vi "Punto 1.vi"() -> ()   [LabVIEW 2020]
panel:
  in  "Operate fuction":bool
  out "C":dbl
  out "B":dbl
  out "A":dbl
  in  "Fuction:":string
  out "X value 1":dbl
  out "X value 2":dbl
  in  "Parar\naplicación":bool
  in  "Parar\naplicación":bool
  out "X value":dbl
  in  "Operate 4y^2-(2z/3)":bool
  in  "Operate 2y^3 + v(10z)":bool
  in  "Operate 44y - 21 z":bool
  in  "Operate 2y + 10z":bool
  in  "Z number":dbl
  in  "Y number":dbl
  # "This program was created by Juan Bermúdez from the Army Aviation School\nat the Aircraft Engineering of the assignature of Programation II"
  # "How to write the fuction?:\n1- First write all in lower case.\n2- Second, write every coefficient, even if this is 0 or 1.\n3- Third, write without spaces.\n4- Forth, write only the necesary things, coming up, some examples:\n\n- 1x^2+2x+3\n- 3x^2-0x+1\n- -4x^2+1x+0\n- -1x^2-10x-9\n The before examples are the correct way to write the fuction."
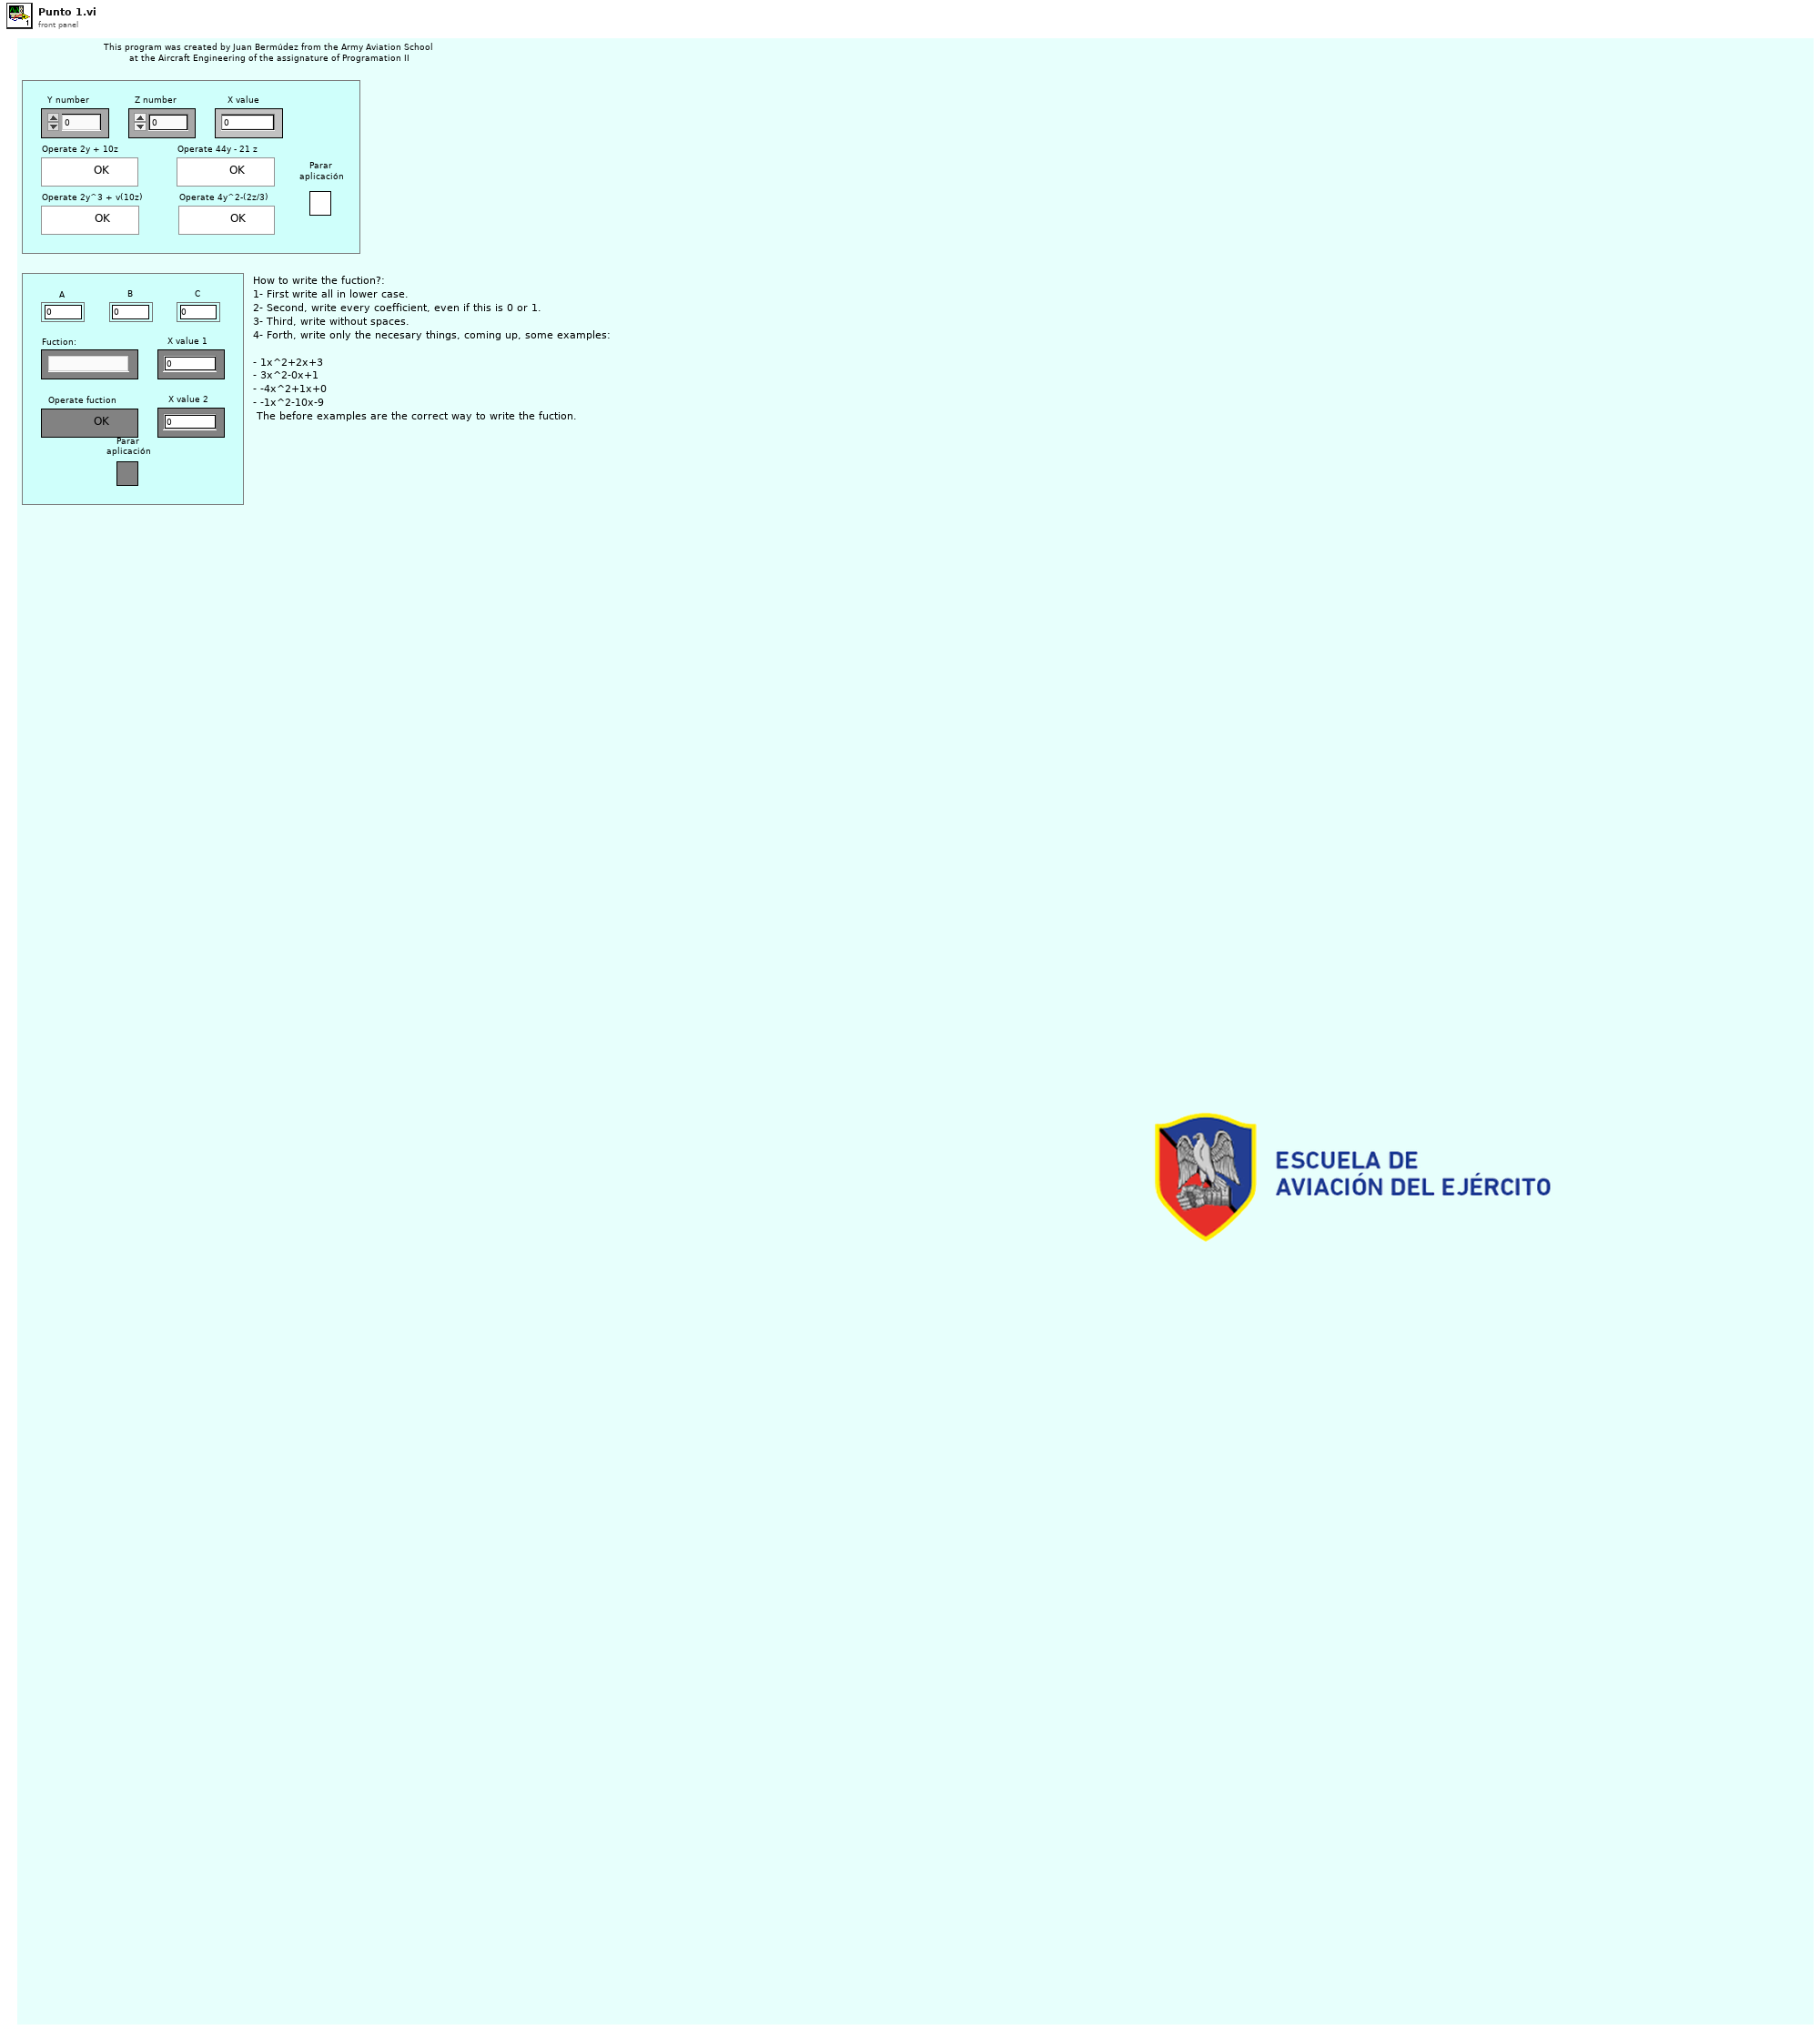
[diagram p1: front panel]
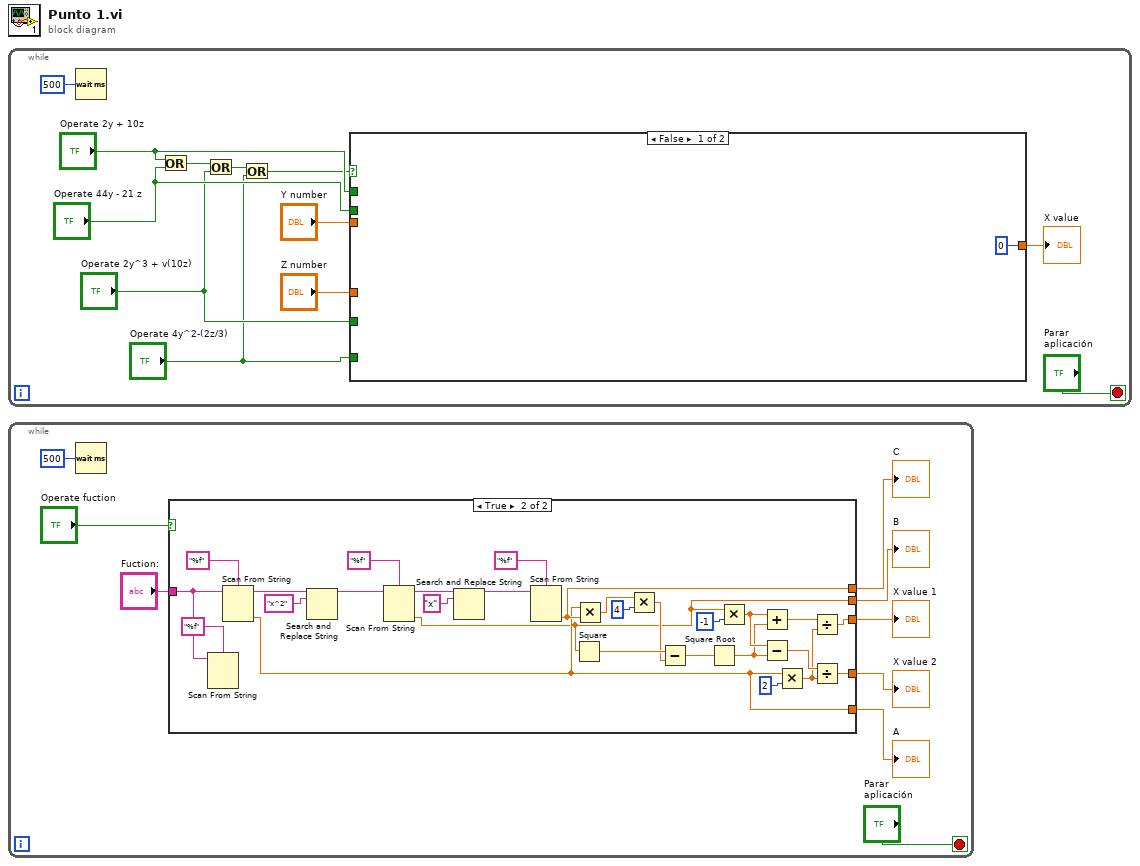
[diagram p0: block diagram]
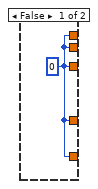
[diagram p2: hidden frame]
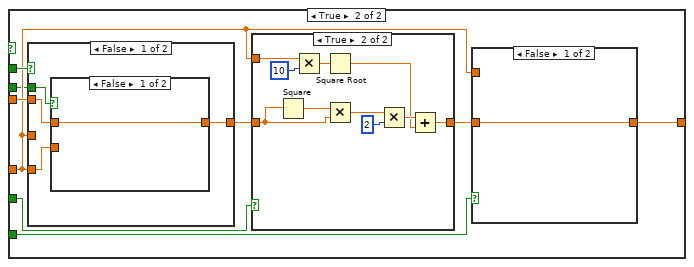
[diagram p3: hidden frame]
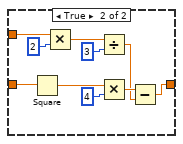
[diagram p4: hidden frame]
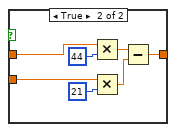
[diagram p6: hidden frame]
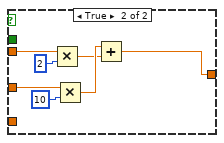
[diagram p7: hidden frame]
diagram:
  n1 = while {
    stop <- "Parar\naplicación" stop-if-true
    n2 = Wait (ms)(milliseconds to wait=500) -> ()  [unwired: 1 out]
    n3 = Or(x="Operate 2y + 10z", y="Operate 44y - 21 z") -> (x .or. y?=w5:bool)
    n4 = Or(x=w5, y="Operate 2y^3 + v(10z)") -> (x .or. y?=w3:bool)
    n5 = Or(x=w3, y="Operate 4y^2-(2z/3)") -> (x .or. y?=w1:bool)
    n6 = case shown="False" w1 {
      tunnel: "Operate 2y + 10z" -> [_ w22]
      tunnel: "Y number" -> [_ w21]
      tunnel: "Operate 2y^3 + v(10z)" -> [_ w20]
      tunnel: "Operate 4y^2-(2z/3)" -> [_ w19]
      tunnel: [0 w17] -> w11
      tunnel: "Z number" -> [_ w16]
      tunnel: "Operate 44y - 21 z" -> [_ w14]
      frame False {
      }
      frame True {
        n7 = case shown="False" w22 {
          tunnel: w16 -> [_ w61]
          tunnel: w21 -> [w46 w63]
          tunnel: w16 -> [w48 _]
          tunnel: [w47 w57] -> w15
          tunnel: w14 -> [w45 _]
          frame False {
            n8 = case shown="False" w45 {
              tunnel: w46 -> [w49 w56]
              tunnel: w48 -> [_ w54]
              tunnel: [w49 w50] -> w47
              frame False {
              }
              frame True {
                n9 = Multiply(x=w56, y=44) -> (x*y=w52:dbl)
                n10 = Multiply(x=w54, y=21) -> (x*y=w51:dbl)
                n11 = Subtract(x=w52, y=w51) -> (x-y=w50:dbl)
              }
            }
          }
          frame True {
            n12 = Multiply(x=w63, y=2) -> (x*y=w58:dbl)
            n13 = Multiply(x=w61, y=10) -> (x*y=w59:dbl)
            n14 = Add(x=w59, y=w58) -> (x+y=w57:dbl)
          }
        }
        n15 = case shown="True" w20 {
          tunnel: w15 -> [w34 w43]
          tunnel: w16 -> [_ w40]
          tunnel: [w34 w35] -> w18
          frame False {
          }
          frame True {
            n16 = Square(x=w43) -> (x^2=w44:dbl)
            n17 = Multiply(x=w40, y=10) -> (x*y=w38:dbl)
            n18 = Square Root(x=w38) -> (sqrt(x)=w36:dbl)
            n19 = Multiply(x=w44, y=w43) -> (x*y=w42:dbl)
            n20 = Multiply(x=w42, y=2) -> (x*y=w37:dbl)
            n21 = Add(x=w37, y=w36) -> (x+y=w35:dbl)
          }
        }
        n22 = case shown="False" w19 {
          tunnel: w18 -> [w23 w33]
          tunnel: w16 -> [_ w30]
          tunnel: [w23 w24] -> w17
          frame False {
          }
          frame True {
            n23 = Square(x=w33) -> (x^2=w32:dbl)
            n24 = Multiply(x=w30, y=2) -> (x*y=w28:dbl)
            n25 = Divide(x=w28, y=3) -> (x/y=w25:dbl)
            n26 = Multiply(x=w32, y=4) -> (x*y=w26:dbl)
            n27 = Subtract(x=w26, y=w25) -> (x-y=w24:dbl)
          }
        }
      }
    }
    "X value" <- w11
  }
  n28 = while {
    stop <- "Parar\naplicación" stop-if-true
    n29 = Wait (ms)(milliseconds to wait=500) -> ()  [unwired: 1 out]
    n30 = case shown="True" "Operate fuction" {
      tunnel: [w73 w89] -> w70
      tunnel: [w73 w88] -> w69
      tunnel: "Fuction:" -> [_ w75]
      tunnel: [w73 w78] -> w67
      tunnel: [w73 w77] -> w66
      tunnel: [w73 w76] -> w65
      frame False {
        w73 = 0
      }
      frame True {
        n31 = Scan From String(format string="%f", input string=w75) -> ()  [unwired: 4 in, 3 out]
        n32 = Scan From String(format string="%f", input string=w75) -> (remaining string=w86:string, output 1=w77:dbl)  [unwired: 3 in, 2 out]
        n33 = Search and Replace String(input string=w86, search string="x^2") -> (result string=w84:string)  [unwired: 6 in, 3 out]
        n34 = Scan From String(format string="%f", input string=w84) -> (remaining string=w82:string, output 1=w76:dbl)  [unwired: 3 in, 2 out]
        n35 = Search and Replace String(input string=w82, search string="x") -> (result string=w80:string)  [unwired: 6 in, 3 out]
        n36 = Scan From String(format string="%f", input string=w80) -> (output 1=w78:dbl)  [unwired: 3 in, 3 out]
        n37 = Square(x=w76) -> (x^2=w99:dbl)
        n38 = Multiply(x=w77, y=w78) -> (x*y=w101:dbl)
        n39 = Multiply(x=w101, y=4) -> (x*y=w98:dbl)
        n40 = Subtract(x=w99, y=w98) -> (x-y=w97:dbl)
        n41 = Square Root(x=w97) -> (sqrt(x)=w94:dbl)
        n42 = Multiply(x=w76, y=-1) -> (x*y=w95:dbl)
        n43 = Add(x=w95, y=w94) -> (x+y=w92:dbl)
        n44 = Subtract(x=w95, y=w94) -> (x-y=w91:dbl)
        n45 = Multiply(x=w77, y=2) -> (x*y=w90:dbl)
        n46 = Divide(x=w92, y=w90) -> (x/y=w89:dbl)
        n47 = Divide(x=w91, y=w90) -> (x/y=w88:dbl)
      }
    }
    "X value 2" <- w69
    "X value 1" <- w70
    "A" <- w66
    "B" <- w65
    "C" <- w67
  }
